vi "RT_MATH_RMS.vi"(8 "Data_In":sgl, 9 "Sample_No":sgl=60.0, 10 "RMS_En":bool, 11 "Array_In":sgl[](array[numeric])) -> (0 "Data_Out":sgl, 3 "Array_Out":sgl[](array[numeric]))   [LabVIEW 2024]
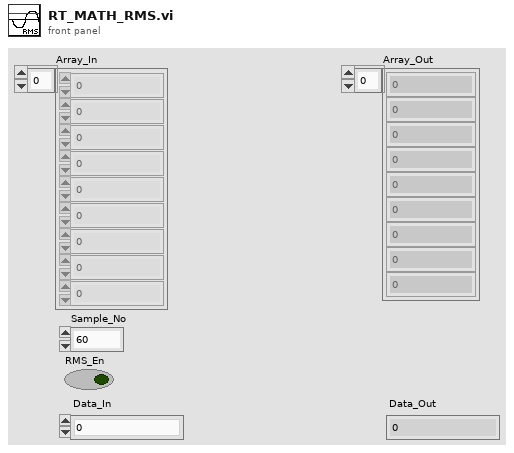
[diagram p1: front panel]
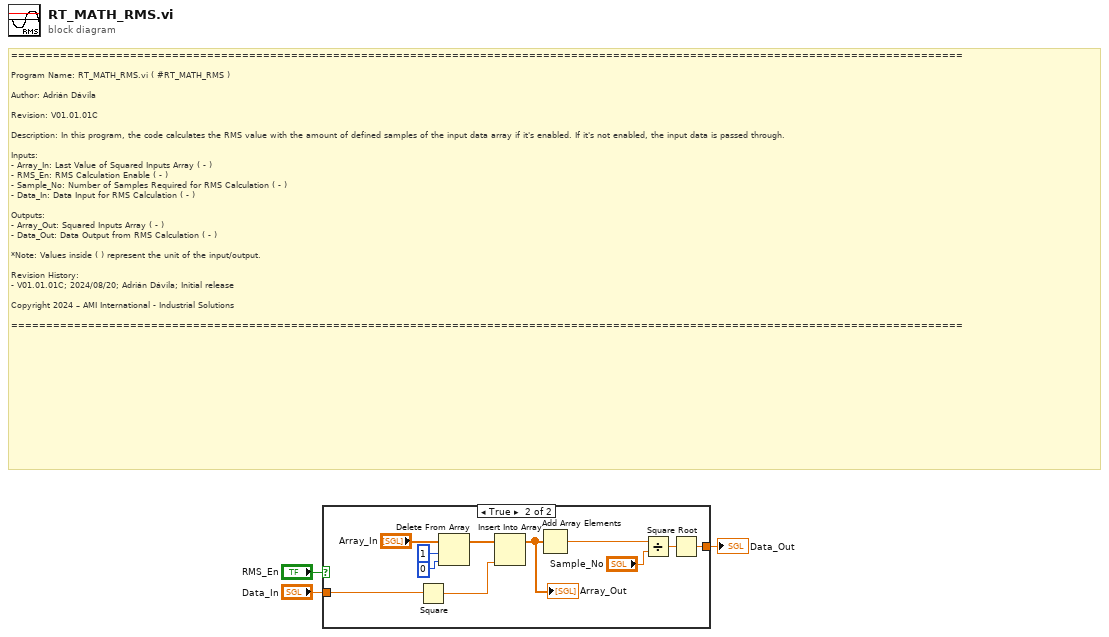
[diagram p0: block diagram]
diagram:
  # "========================================================================================================================================\n\nProgram Name: RT_MATH_RMS.vi ( #RT_MATH_RMS )\n\nAuthor: Adrián Dávila\n\nRevision: V01.01.01C\n\nDescription: In this program, the code calculates the RMS value with the amount of defined samples of the input data array if it's enabled. If it's not enabled, the input data is passed through. \n\nInputs:\n- Array_In: Last Value of Squared Inputs Array ( - )\n- RMS_En: RMS Calculation Enable ( - ) \n- Sample_No: Number of Samples Required for RMS Calculation ( - )\n- Data_In: Data Input for RMS Calculation ( - )\n\nOutputs:\n- Array_Out: Squared Inputs Array ( - )\n- Data_Out: Data Output from RMS Calculation ( - )\n\n*Note: Values inside ( ) represent the unit of the input/output.\n \nRevision History:\n- V01.01.01C; 2024/08/20; Adrián Dávila; Initial release\n\nCopyright 2024 – AMI International - Industrial Solutions\n\n========================================================================================================================================"
  n1 = case shown="True" "RMS_En" {
    tunnel: "Data_In" -> [w4 w7]
    tunnel: [w4 w5] -> w3
    frame False {
    }
    frame True {
      n2 = Square(x=w7) -> (x^2=w10:sgl)
      n3 = Delete From Array(array="Array_In", length=1, index=0) -> (array with subset deleted=w12:sgl[])  [unwired: 1 out]
      n4 = Insert Into Array(array=w12, new element=w10) -> (w11:sgl[])  [unwired: 1 in]
      "Array_Out" <- w11
      n5 = Add Array Elements(numeric array=w11) -> (sum=w9:sgl)
      n6 = Divide(x=w9, y="Sample_No") -> (x/y=w8:sgl)
      n7 = Square Root(x=w8) -> (sqrt(x)=w5:sgl)
    }
  }
  "Data_Out" <- w3
